vi "run_database.vi"() -> ()   [LabVIEW 2011]
uses:
  <vilib>/addons/database/Connection.llb/DB Tools Open Connec (String).vi
  databasePath.vi
  <vilib>/addons/database/NI_Database_API.lvlib
panel:
  out "Connection Error 3":errorcluster
  out "Received Data from counter.vi":string
  out "# Received Data from counter.vi":u64
  out "Dequeue Rate (per second)":dbl
  out "# Elements in Real-time Queue":u64
  out "# Received Data from plc.vi":u64
  out "Connection Error 2":errorcluster
  out "Received Data from plc.vi":string
  out "# of Dequeues (total)":u64
  in  "Pause Database Writing (s)":dbl=5.0
  in  "Backup Interval (hour)":dbl=10.0
  out "Backup Error Msg":string
  out "Database Backup Path":path
  out "Dequeue Paused":bool
  out "# of Backups":u64
  out "Next Backup Dues in (s):":u64 caption="Elapsed Time (s)"
  out "Database Path":path
  out "cmd string for sqlite3.exe":string
  out "# Elements in Database Queue":u64
  out "Received Data from mote.vi":string
  out "Dequeue Error":errorcluster
  out "Database Access Error":errorcluster
  out "# Received Data from mote.vi":u64
  out "Connection Error":errorcluster
  # "Receive data from motes and Enqueue"
  # "Dequeue and write to database"
  # "Backup database"
  # "Receive data from plcs and Enqueue"
  # "Receive data from people counter and Enqueue"
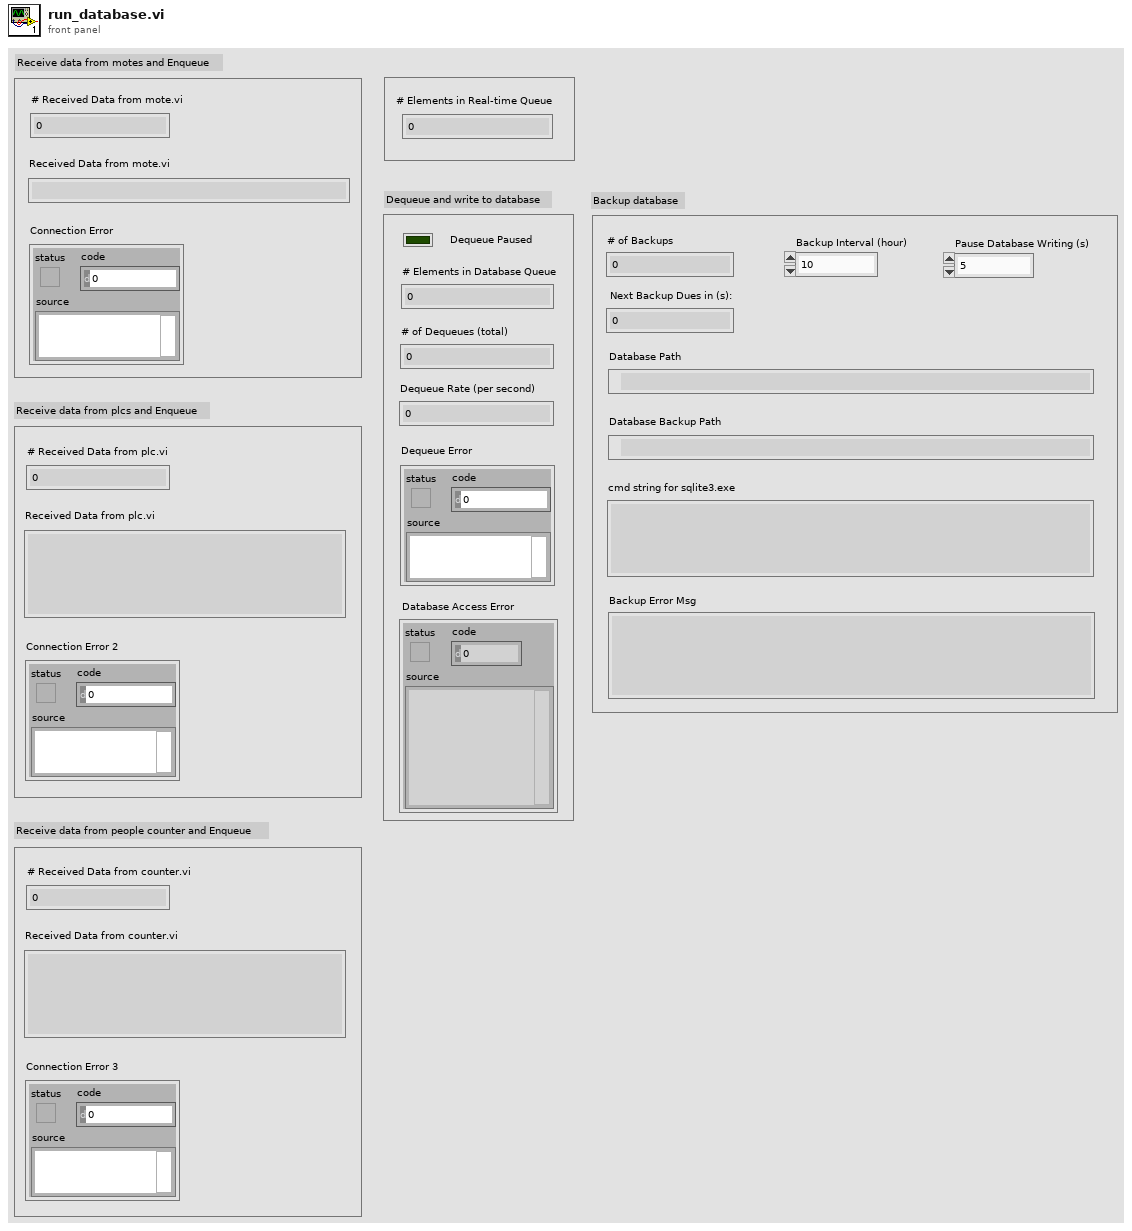
[diagram p1: front panel]
types:
  T1 = enum16{"Read", "Write", "ReadWrite", "BufferedRead", "BufferedReadWrite"}
  T2 = cluster{string, string, string, string, string, string}
  T3 = cluster{string, "output string":string, "output string":string, "output string":string, "output string":string, "output string":string}
  T4 = cluster{string, "data 1 (2 bytes)":u16, "data 2 (2 bytes)":u16, "data 3 (2 bytes)":u16, "data 4 (2 bytes)":u16, "Timestamp (19 bytes)":string, "location":string}
  T5 = cluster{string, string, string, string, "Timestamp (19 bytes)":string, "location":string}
  T6 = typedef "NI_Database_API.lvlib/Conn ObjectReference.ctl" = refnum<k1>
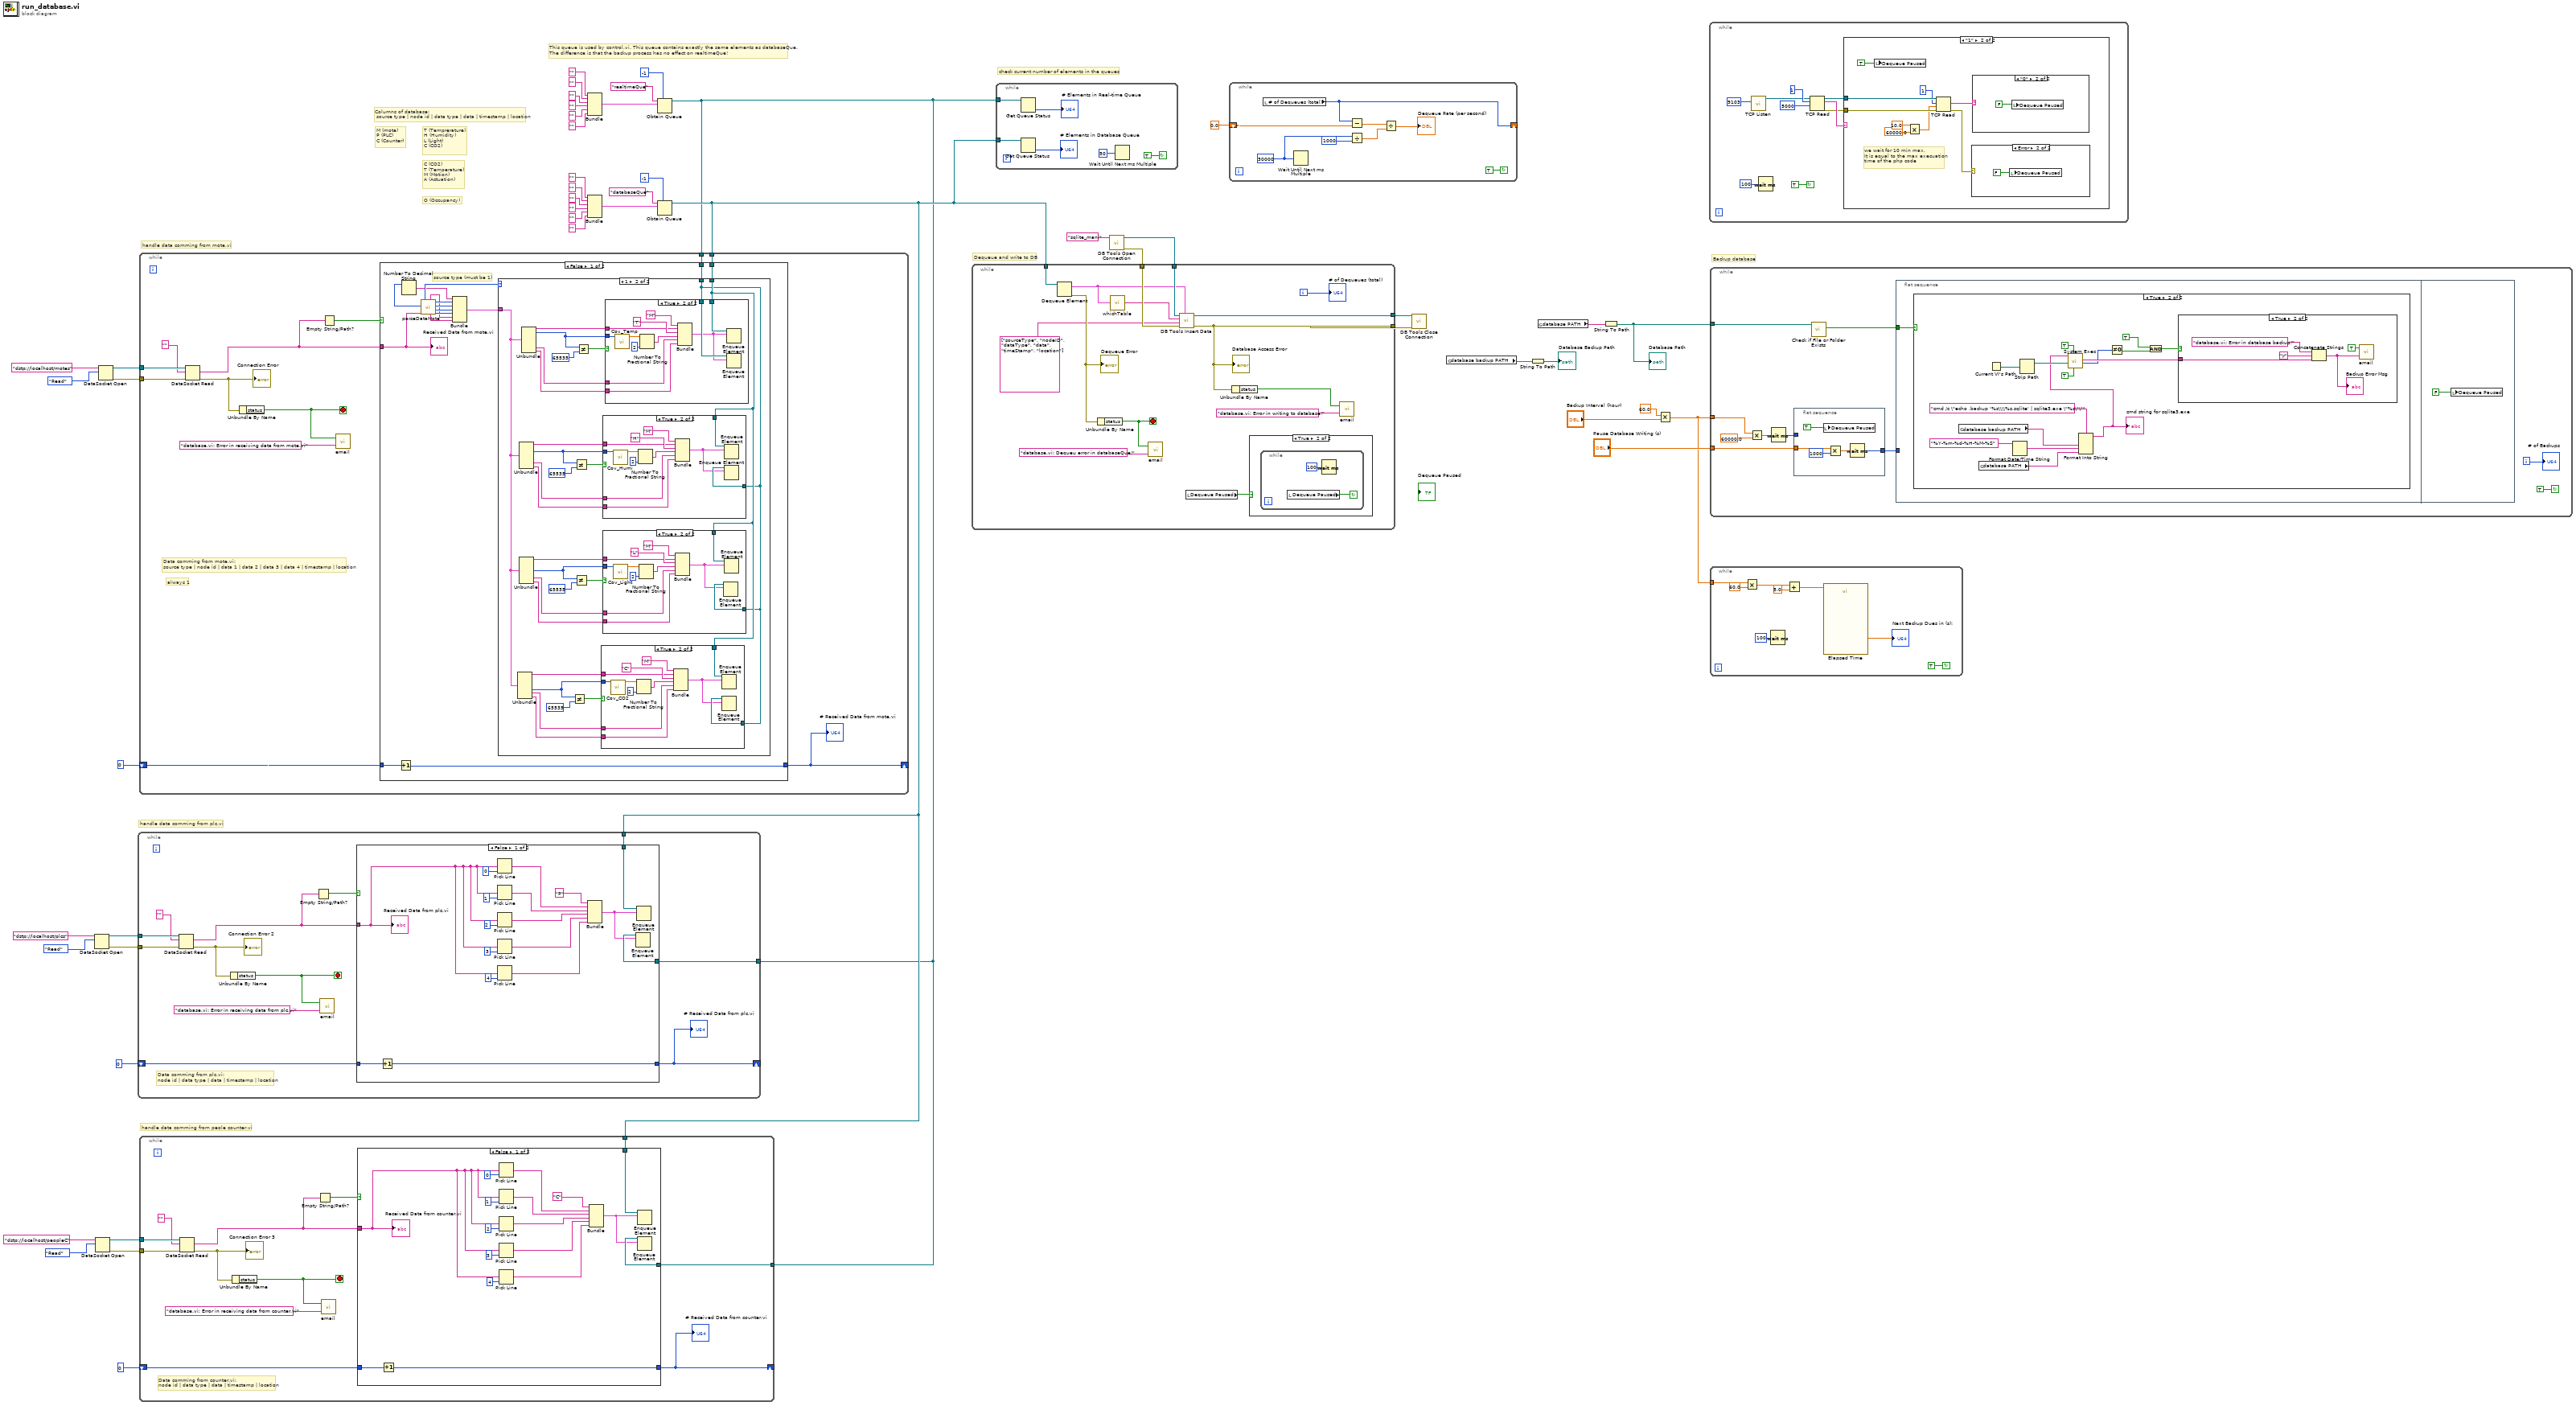
[diagram p0: block diagram]
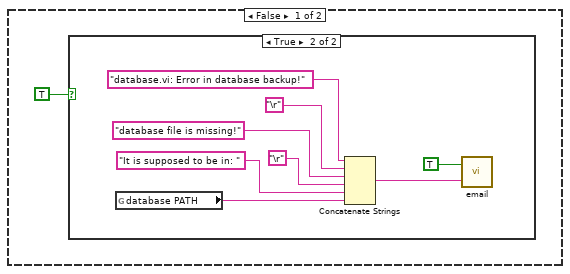
[diagram p7: hidden frame]
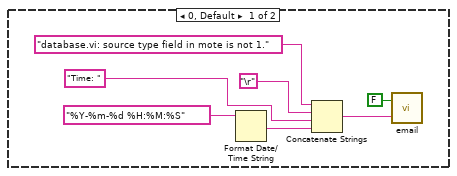
[diagram p11: hidden frame]
diagram:
  # "handle data comming from peole counter.vi"
  # "O (Occupancy)"
  # "C (CO2)\nT (Temperature)\nM (Motion)\nA (Actuation)"
  # "This queue is used by control.vi. This queue contains exactly the same elements as databaseQue.\nThe difference is that the backup process has no effect on realtimeQue!"
  # "handle data comming from plc.vi"
  # "handle data comming from mote.vi"
  # "Backup database"
  # "Dequeue and write to DB"
  # "check current number of elements in the queues"
  # "M (mote)\nP (PLC)\nC (Counter)"
  # "T (Temprerature)\nH (Humidity)\nL (Light)\nC (CO2)"
  # "Columns of database:\n source type | node id | data type | data | timestamp | location"
  n1 = DataSocket Open(10:T1."Read" ("mode"), 11:"dstp://localhost/plcs" ("URL 3")) -> (0:w27:errorcluster, 3:w26:refnum<k13>)  [unwired: 2 in]
  n2 = DataSocket Open(10:T1."Read" ("mode"), 11:"dstp://localhost/peopleC" ("URL 3")) -> (0:w9:errorcluster, 3:w10:refnum<k13>)  [unwired: 2 in]
  n3 = DataSocket Open(10:T1."Read" ("mode"), 11:"dstp://localhost/motes" ("URL 3")) -> (0:w31:errorcluster, 3:w30:refnum<k13>)  [unwired: 2 in]
  n4 = Bundle("", "", "", "", "", "") -> (w21:T2)  [unwired: 1 in]
  n5 = Bundle("", "", "", "", "", "") -> (w42:T2)  [unwired: 1 in]
  n6 = Obtain Queue(max queue size (-1, unlimited)=-1, name (unnamed)="realtimeQue", element data type=w21) -> (queue out=w5:refnum<queue>)  [unwired: 2 in, 2 out]
  n7 = Obtain Queue(max queue size (-1, unlimited)=-1, name (unnamed)="databaseQue", element data type=w42) -> (queue out=w6:refnum<queue>)  [unwired: 2 in, 2 out]
  n8 = while {
    tunnel: w27 -> [w61]
    tunnel: w26 -> [w60]
    tunnel: w6 -> [w58]
    tunnel: w5 -> [w56]
    shift-right: [w51] -> _
    shift-left: u64 0 -> [w52]
    stop <- w53 stop-if-true
    # "Data comming from plc.vi:\nnode id | data type | data | timestamp | location"
    n9 = DataSocket Read(8:w61, 10:"", 11:w60) -> (0:w59:errorcluster, 2:w54:string)  [unwired: 2 in, 5 out]
    "Connection Error 2" <- w59
    n10 = Unbundle By Name(w59) -> ("status"=w53:bool)
    n11 = Empty String/Path?(string/path=w54) -> (empty?=w55:bool)
    n12 = call "email.vi"("Body"="database.vi: Error in receiving data from plc.vi", "Enable"=w53) -> ()  [unwired: 1 in]
    n13 = case shown="False" w55 {
      tunnel: w58 -> [w78 _]
      tunnel: w54 -> [w67 _]
      tunnel: w56 -> [w66 _]
      tunnel: w52 -> [w63 w79]
      tunnel: [w62 w79] -> w51
      frame False {
        n14 = Increment(x=w63) -> (x+1=w62:u64)
        n15 = Pick Line(multi-line string=w67, line index=0) -> (output string=w68:string)  [unwired: 1 in]
        n16 = Pick Line(multi-line string=w67, line index=1) -> (output string=w71:string)  [unwired: 1 in]
        n17 = Pick Line(multi-line string=w67, line index=2) -> (output string=w64:string)  [unwired: 1 in]
        n18 = Pick Line(multi-line string=w67, line index=3) -> (output string=w70:string)  [unwired: 1 in]
        n19 = Pick Line(multi-line string=w67, line index=4) -> (output string=w69:string)  [unwired: 1 in]
        n20 = Bundle("P", "output string"=w68, "output string"=w71, "output string"=w64, "output string"=w70, "output string"=w69) -> (w65:T3)  [unwired: 1 in]
        n21 = Enqueue Element(queue=w66, element=w65) -> ()  [unwired: 2 in, 3 out]
        n22 = Enqueue Element(queue=w78, element=w65) -> ()  [unwired: 2 in, 3 out]
        "Received Data from plc.vi" <- w67
      }
      frame True {
      }
    }
    "# Received Data from plc.vi" <- w51
  }
  n23 = while {
    tunnel: w31 -> [w91]
    tunnel: w30 -> [w90]
    tunnel: w6 -> [w88]
    tunnel: w5 -> [w86]
    shift-right: [w81] -> _
    shift-left: u64 0 -> [w82]
    stop <- w83 stop-if-true
    # "Data comming from mote.vi:\nsource type | node id | data 1 | data 2 | data 3 | data 4 | timestamp | location"
    # "always 1"
    n24 = DataSocket Read(8:w91, 10:"", 11:w90) -> (0:w89:errorcluster, 2:w84:string)  [unwired: 2 in, 5 out]
    "Connection Error" <- w89
    n25 = Unbundle By Name(w89) -> ("status"=w83:bool)
    n26 = Empty String/Path?(string/path=w84) -> (empty?=w85:bool)
    n27 = call "email.vi"("Body"="database.vi: Error in receiving data from mote.vi", "Enable"=w83) -> ()  [unwired: 1 in]
    n28 = case shown="False" w85 {
      tunnel: w88 -> [w98 _]
      tunnel: w84 -> [w95 _]
      tunnel: w86 -> [w94 _]
      tunnel: [w93 w189] -> w81
      tunnel: w82 -> [w92 w189]
      frame False {
        # "source type (must be 1)"
        n29 = Increment(x=w92) -> (x+1=w93:u64)
        n30 = call "parseDataMote.vi"("input data"=w95) -> ("source type (1 byte)"=w105:u8, "node id (1 byte)"=w97:u8, "Timestamp (19 bytes)"=w100:string, "location"=w99:string, "data 1 (2 bytes)"=w104:u16, "data 2 (2 bytes)"=w103:u16, "data 3 (2 bytes)"=w102:u16, "data 4 (2 bytes)"=w101:u16)  [unwired: 1 in]
        n31 = Number To Decimal String(number=w97) -> (decimal integer string=w96:string)  [unwired: 1 in]
        n32 = Bundle(w96, "data 1 (2 bytes)"=w104, "data 2 (2 bytes)"=w103, "data 3 (2 bytes)"=w102, "data 4 (2 bytes)"=w101, "Timestamp (19 bytes)"=w100, "location"=w99) -> (w106:T4)  [unwired: 1 in]
        n33 = case shown="1" w105 {
          tunnel: w106 -> [_ w119]
          tunnel: w98 -> [_ w115]
          tunnel: w94 -> [_ w114]
          frame 0, Default {
            n34 = Format Date/Time String(time format string (%c)="%Y-%m-%d %H:%M:%S") -> (date/time string=w109:string)  [unwired: 2 in]
            n35 = Concatenate Strings("database.vi: source type field in mote is not 1.", "\r", "Time: ", w109) -> (w110:string)
            n36 = call "email.vi"("Body"=w110, "Enable"=FALSE) -> ()  [unwired: 1 in]
          }
          frame 1 {
            n37 = Unbundle(w119) -> (w122:string, "data 4 (2 bytes)"=w116:u16, "Timestamp (19 bytes)"=w121:string, "location"=w120:string)  [unwired: 3 out]
            n38 = Unbundle(w119) -> (w132:string, "data 2 (2 bytes)"=w118:u16, "Timestamp (19 bytes)"=w131:string, "location"=w130:string)  [unwired: 3 out]
            n39 = Unbundle(w119) -> (w127:string, "data 3 (2 bytes)"=w117:u16, "Timestamp (19 bytes)"=w126:string, "location"=w125:string)  [unwired: 3 out]
            n40 = Unbundle(w119) -> (w138:string, "data 1 (2 bytes)"=w137:u16, "Timestamp (19 bytes)"=w136:string, "location"=w135:string)  [unwired: 3 out]
            n41 = Not Equal?(x=w116, y=u16 65535) -> (x != y?=w124:bool)
            n42 = Not Equal?(x=w118, y=u16 65535) -> (x != y?=w134:bool)
            n43 = Not Equal?(x=w117, y=u16 65535) -> (x != y?=w129:bool)
            n44 = Not Equal?(x=w137, y=u16 65535) -> (x != y?=w140:bool)
            n45 = case shown="True" w124 {
              tunnel: w122 -> [_ w150]
              tunnel: w116 -> [_ w149]
              tunnel: w121 -> [_ w148]
              tunnel: w120 -> [_ w147]
              tunnel: w115 -> [_ w146]
              tunnel: w114 -> [_ w145]
              frame False {
              }
              frame True {
                n46 = call "Cov_CO2.vi"("Input x"=w149) -> ("CO2"=w143:dbl)  [unwired: 10 in]
                n47 = Number To Fractional String(number=w143, precision (6)=i16 2) -> (F-format string=w142:string)  [unwired: 2 in]
                n48 = Bundle("M", w150, "C", w142, "Timestamp (19 bytes)"=w148, "location"=w147) -> (w144:T5)  [unwired: 1 in]
                n49 = Enqueue Element(queue=w145, element=w144) -> ()  [unwired: 2 in, 3 out]
                n50 = Enqueue Element(queue=w146, element=w144) -> ()  [unwired: 2 in, 3 out]
              }
            }
            n51 = case shown="True" w134 {
              tunnel: w132 -> [_ w174]
              tunnel: w118 -> [_ w173]
              tunnel: w131 -> [_ w172]
              tunnel: w130 -> [_ w171]
              tunnel: w115 -> [_ w170]
              tunnel: w114 -> [_ w169]
              frame False {
              }
              frame True {
                n52 = call "Cov_Humi.vi"("Input x"=w173) -> ("Humidity"=w167:dbl)  [unwired: 10 in]
                n53 = Number To Fractional String(number=w167, precision (6)=i16 2) -> (F-format string=w166:string)  [unwired: 2 in]
                n54 = Bundle("M", w174, "H", w166, "Timestamp (19 bytes)"=w172, "location"=w171) -> (w168:T5)  [unwired: 1 in]
                n55 = Enqueue Element(queue=w170, element=w168) -> ()  [unwired: 2 in, 3 out]
                n56 = Enqueue Element(queue=w169, element=w168) -> ()  [unwired: 2 in, 3 out]
              }
            }
            n57 = case shown="True" w129 {
              tunnel: w127 -> [_ w162]
              tunnel: w117 -> [_ w158]
              tunnel: w126 -> [_ w161]
              tunnel: w125 -> [_ w160]
              tunnel: w115 -> [_ w159]
              tunnel: w114 -> [_ w157]
              frame False {
              }
              frame True {
                n58 = call "Cov_Light.vi"("Input x"=w158) -> ("Light"=w155:dbl)  [unwired: 10 in]
                n59 = Number To Fractional String(number=w155, precision (6)=i16 2) -> (F-format string=w154:string)  [unwired: 2 in]
                n60 = Bundle("M", w162, "L", w154, "Timestamp (19 bytes)"=w161, "location"=w160) -> (w156:T5)  [unwired: 1 in]
                n61 = Enqueue Element(queue=w157, element=w156) -> ()  [unwired: 2 in, 3 out]
                n62 = Enqueue Element(queue=w159, element=w156) -> ()  [unwired: 2 in, 3 out]
              }
            }
            n63 = case shown="True" w140 {
              tunnel: w138 -> [_ w186]
              tunnel: w137 -> [_ w185]
              tunnel: w136 -> [_ w184]
              tunnel: w135 -> [_ w183]
              tunnel: w115 -> [_ w182]
              tunnel: w114 -> [_ w181]
              frame False {
              }
              frame True {
                n64 = call "Cov_Temp.vi"("Input x"=w185) -> ("Temperature"=w179:dbl)  [unwired: 10 in]
                n65 = Number To Fractional String(number=w179, precision (6)=i16 2) -> (F-format string=w178:string)  [unwired: 2 in]
                n66 = Bundle("M", w186, "T", w178, "Timestamp (19 bytes)"=w184, "location"=w183) -> (w180:T5)  [unwired: 1 in]
                n67 = Enqueue Element(queue=w182, element=w180) -> ()  [unwired: 2 in, 3 out]
                n68 = Enqueue Element(queue=w181, element=w180) -> ()  [unwired: 2 in, 3 out]
              }
            }
          }
        }
        "Received Data from mote.vi" <- w95
      }
      frame True {
      }
    }
    "# Received Data from mote.vi" <- w81
  }
  n69 = while {
    tunnel: w9 -> [w201]
    tunnel: w10 -> [w200]
    tunnel: w6 -> [w198]
    tunnel: w5 -> [w196]
    shift-right: [w191] -> _
    shift-left: u64 0 -> [w192]
    stop <- w193 stop-if-true
    # "Data comming from counter.vi:\nnode id | data type | data | timestamp | location"
    n70 = DataSocket Read(8:w201, 10:"", 11:w200) -> (0:w199:errorcluster, 2:w194:string)  [unwired: 2 in, 5 out]
    "Connection Error 3" <- w199
    n71 = Unbundle By Name(w199) -> ("status"=w193:bool)
    n72 = Empty String/Path?(string/path=w194) -> (empty?=w195:bool)
    n73 = call "email.vi"("Body"="database.vi: Error in receiving data from counter.vi", "Enable"=w193) -> ()  [unwired: 1 in]
    n74 = case shown="False" w195 {
      tunnel: w198 -> [w218 _]
      tunnel: w194 -> [w207 _]
      tunnel: w196 -> [w206 _]
      tunnel: w192 -> [w203 w219]
      tunnel: [w202 w219] -> w191
      frame False {
        n75 = Increment(x=w203) -> (x+1=w202:u64)
        n76 = Pick Line(multi-line string=w207, line index=0) -> (output string=w208:string)  [unwired: 1 in]
        n77 = Pick Line(multi-line string=w207, line index=1) -> (output string=w211:string)  [unwired: 1 in]
        n78 = Pick Line(multi-line string=w207, line index=2) -> (output string=w204:string)  [unwired: 1 in]
        n79 = Pick Line(multi-line string=w207, line index=3) -> (output string=w210:string)  [unwired: 1 in]
        n80 = Pick Line(multi-line string=w207, line index=4) -> (output string=w209:string)  [unwired: 1 in]
        n81 = Bundle("C", "output string"=w208, "output string"=w211, "output string"=w204, "output string"=w210, "output string"=w209) -> (w205:T3)  [unwired: 1 in]
        n82 = Enqueue Element(queue=w206, element=w205) -> ()  [unwired: 2 in, 3 out]
        n83 = Enqueue Element(queue=w218, element=w205) -> ()  [unwired: 2 in, 3 out]
        "Received Data from counter.vi" <- w207
      }
      frame True {
      }
    }
    "# Received Data from counter.vi" <- w191
  }
  n84 = while {
    tunnel: w6 -> [w225]
    tunnel: w5 -> [w221]
    stop <- TRUE continue-if-true
    n85 = Get Queue Status(queue=w225) -> (# elements in queue=→"# Elements in Database Queue":i32)  [unwired: 2 in, 7 out]
    n86 = Get Queue Status(queue=w221) -> (# elements in queue=→"# Elements in Real-time Queue":i32)  [unwired: 2 in, 7 out]
    n87 = Wait Until Next ms Multiple(millisecond multiple=u32 50) -> ()  [unwired: 1 out]
  }
  n88 = call-poly <vilib>:"DB Tools Open Connection.vi"("connection information"="sqlite_mani") -> ("error out"=w37:errorcluster, "connection reference"=w43:T6)  [unwired: 7 in]
  n89 = while {
    tunnel: w43 -> [w239]
    tunnel: [w240] -> w39
    tunnel: [w229] -> w38
    tunnel: w37 -> [w238]
    tunnel: w6 -> [w237]
    i -> [w233]
    stop <- w230 stop-if-true
    n90 = Dequeue Element(queue=w237) -> (element=w231:T2, error out=w236:errorcluster)  [unwired: 2 in, 2 out]
    "Dequeue Error" <- w236
    n91 = Unbundle By Name(w236) -> ("status"=w230:bool)
    n92 = call "whichTable.vi"("element"=w231) -> ("String"=w232:string)
    n93 = call "email.vi"("Body"="database.vi: Dequeu error in databaseQue!", "Enable"=w230) -> ()  [unwired: 1 in]
    n94 = call <vilib>:"DB Tools Insert Data.vi"("data"=w231, "error in (no error)"=w238, "columns"=string[] ["sourceType", "nodeID", "dataType", "data", "timeStamp", "location"], "table"=w232, "connection reference"=w239) -> ("error out"=w229:errorcluster, "connection reference out"=w240:T6)  [unwired: 5 in]
    "Database Access Error" <- w229
    n95 = local read "Dequeue Paused"() -> (w234:bool)
    n96 = Unbundle By Name(w229) -> ("status"=w228:bool)
    n97 = case shown="True" w234 {
      frame False {
      }
      frame True {
        n98 = while {
          stop <- w241 continue-if-true
          n99 = local read "Dequeue Paused"() -> (w241:bool)
          n100 = Wait (ms)(milliseconds to wait=u32 100) -> ()  [unwired: 1 out]
        }
      }
    }
    n101 = call "email.vi"("Body"="database.vi: Error in writing to database!", "Enable"=w228) -> ()  [unwired: 1 in]
    "# of Dequeues (total)" <- w233
  }
  n102 = while {
    shift-right: [w248] -> _
    shift-left: 0.0 -> [w249]
    stop <- TRUE continue-if-true
    w245 = u32 30000 ("millisecond multiple")
    n103 = local read "# of Dequeues (total)"() -> (w248:u64)
    n104 = Wait Until Next ms Multiple(millisecond multiple=w245) -> ()  [unwired: 1 out]
    n105 = Subtract(x=w248, y=w249) -> (x-y=w247:dbl)
    n106 = Divide(x=w245, y=u32 1000) -> (x/y=w243:dbl)
    n107 = Divide(x=w247, y=w243) -> (x/y=→"Dequeue Rate (per second)":dbl)
  }
  n108 = call <vilib>:"DB Tools Close Connection.vi"("error in (no error)"=w38, "connection reference"=w39) -> ()  [unwired: 5 in, 1 out]
  n109 = global read "databasePath.vi" "database backup PATH"() -> (w34:string)
  n110 = String To Path(string=w34) -> (path=→"Database Backup Path":path)
  n111 = global read "databasePath.vi" "database PATH"() -> (w36:string)
  n112 = String To Path(string=w36) -> (path=w35:path)
  "Database Path" <- w35
  n113 = Multiply(x=60.0, y="Backup Interval (hour)") -> (x*y=w1:dbl)
  n114 = while {
    stop <- TRUE continue-if-true
    n115 = call <vilib>:"TCP Listen.vi"("port"=u16 9103) -> ("connection ID"=w254:refnum<k5>)  [unwired: 6 in, 4 out]
    n116 = Wait (ms)(milliseconds to wait=u32 100) -> ()  [unwired: 1 out]
    n117 = TCP Read(connection ID=w254, bytes to read=1, 9:5000 ("timeout ms (25000)")) -> (connection ID out=w252:refnum<k5>, data out=w253:string, error out=w251:errorcluster)  [unwired: 2 in]
    n118 = case shown="\"1\"" w253 {
      tunnel: w252 -> [_ w268]
      tunnel: w251 -> [_ w267]
      frame "0", Default {
      }
      frame "1" {
        # "we wait for 10 min max.\nIt is equal to the max execuation\ntime of the php code"
        n119 = local write "Dequeue Paused"(TRUE ("Backup in Progress")) -> ()
        n120 = Multiply(x=10.0, y=60000.0) -> (x*y=w260:dbl)
        n121 = TCP Read(connection ID=w268, bytes to read=1, error in (no error)=w267, 9:w260) -> (data out=w264:string, error out=w263:errorcluster)  [unwired: 1 in, 1 out]
        n122 = case shown="Error" w263 {
          frame No Error {
          }
          frame Error {
            n123 = local write "Dequeue Paused"(FALSE ("Backup in Progress")) -> ()
          }
        }
        n124 = case shown="\"0\"" w264 {
          frame "1", Default {
          }
          frame "0" {
            n125 = local write "Dequeue Paused"(FALSE ("Backup in Progress")) -> ()
          }
        }
      }
    }
  }
  n126 = while {
    tunnel: w1 -> [w276]
    stop <- TRUE continue-if-true
    n127 = Multiply(x=w276, y=60.0) -> (x*y=w273:dbl)
    n128 = Wait (ms)(milliseconds to wait=u32 100) -> ()  [unwired: 1 out]
    n129 = Add(x=w273, y=5.0) -> (x+y=w274:dbl)
    n130 = call "Elapsed Time"("Time Target (s)"=w274) -> ("Elapsed Time (s)"=→"Next Backup Dues in (s):":dbl)  [unwired: 11 in, 7 out]
  }
  n131 = while {
    tunnel: w35 -> [w287]
    tunnel: w1 -> [w281]
    tunnel: "Pause Database Writing (s)" -> [w280]
    i -> [w279]
    stop <- TRUE continue-if-true
    n132 = Multiply(x=w281, y=60000.0) -> (x*y=w282:dbl)
    n133 = Wait (ms)(milliseconds to wait=w282) -> (millisecond timer value=w286:u32)
    n134 = flat-sequence {
      tunnel: w286 -> [_]
      tunnel: [w293] -> w285
      tunnel: w280 -> [w291]
      frame #0 {
        n135 = local write "Dequeue Paused"(TRUE ("Pause Write to DB")) -> ()
        n136 = Multiply(x=w291, y=u32 1000) -> (x*y=w292:dbl)
        n137 = Wait (ms)(milliseconds to wait=w292) -> (millisecond timer value=w293:u32)
      }
    }
    n138 = call <vilib>:"Check if File or Folder Exists.vi"("path"=w287) -> ("file or folder exists?"=w283:bool)  [unwired: 8 in, 2 out]
    n139 = flat-sequence {
      tunnel: w285 -> [_]
      tunnel: w283 -> [w294]
      frame #0 {
        n140 = case shown="True" w294 {
          frame False {
            n141 = case shown="True" TRUE {
              frame False {
              }
              frame True {
                n142 = global read "databasePath.vi" "database PATH"() -> (w298:string)
                n143 = Concatenate Strings("database.vi: Error in database backup!", "\r", "database file is missing!", "\r", "It is supposed to be in: ", w298) -> (w296:string)
                n144 = call "email.vi"("Body"=w296, "Enable"=TRUE) -> ()  [unwired: 1 in]
              }
            }
          }
          frame True {
            n145 = global read "databasePath.vi" "database backup PATH"() -> (w307:string)
            n146 = global read "databasePath.vi" "database PATH"() -> (w309:string)
            n147 = Current VI's Path() -> (path=w314:path)
            n148 = Format Date/Time String(time format string (%c)="%Y-%m-%d-%H-%M-%S") -> (date/time string=w308:string)  [unwired: 2 in]
            n149 = Strip Path(path=w314) -> (stripped path=w313:path)  [unwired: 1 out]
            n150 = Format Into String(format string="cmd /c \"echo .backup '%s\\\\%s.sqlite' | sqlite3.exe \"%s\"\"", w307, w308, w309) -> (resulting string=w304:string)  [unwired: 2 in, 1 out]
            "cmd string for sqlite3.exe" <- w304
            n151 = call <vilib>:"System Exec.vi"("run minimized? (F)"=TRUE, "wait until completion? (T)"=TRUE, "working directory"=w313, "command line"=w304) -> ("return code"=w311:i32, "standard error"=w312:string)  [unwired: 4 in, 2 out]
            n152 = Not Equal To 0?(x=w311) -> (x != 0?=w310:bool)
            n153 = And(x=TRUE, y=w310) -> (x .and. y?=w318:bool)
            n154 = case shown="True" w318 {
              tunnel: w312 -> [_ w321]
              frame False {
              }
              frame True {
                n155 = Concatenate Strings("database.vi: Error in database backup!", "\r", w321) -> (w319:string)
                "Backup Error Msg" <- w319
                n156 = call "email.vi"("Body"=w319, "Enable"=TRUE) -> ()  [unwired: 1 in]
              }
            }
          }
        }
      }
      frame #1 {
        n157 = local write "Dequeue Paused"(FALSE ("Pause Write to DB")) -> ()
      }
    }
    "# of Backups" <- w279
  }
